vi "Subnet Mask to CIDR Prefix.vi"(7 "address":u32) -> (3 "prefix":i32)   [LabVIEW 2020, in "NI_WFCN.lvlib"]
doc: "Given a subnet mask (e.g. 255.255.255.0), returns its equivalent CIDR prefix (e.g. /24)."
uses:
  <vilib>/net/WFCN/NI_WFCN.lvlib
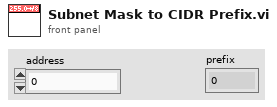
[diagram p1: front panel]
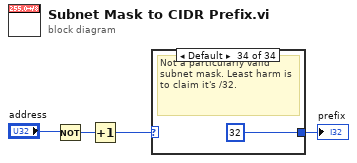
[diagram p0: block diagram]
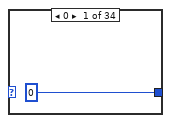
[diagram p2: hidden frame]
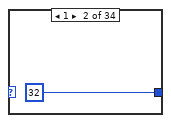
[diagram p3: hidden frame]
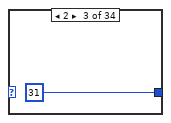
[diagram p4: hidden frame]
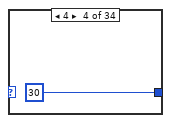
[diagram p5: hidden frame]
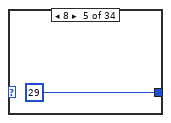
[diagram p6: hidden frame]
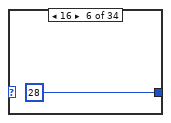
[diagram p7: hidden frame]
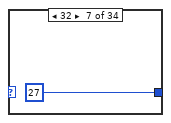
[diagram p8: hidden frame]
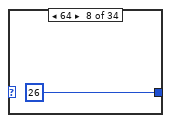
[diagram p9: hidden frame]
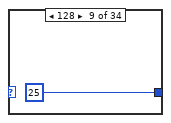
[diagram p10: hidden frame]
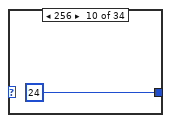
[diagram p11: hidden frame]
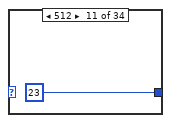
[diagram p12: hidden frame]
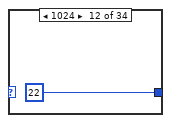
[diagram p13: hidden frame]
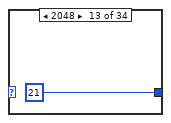
[diagram p14: hidden frame]
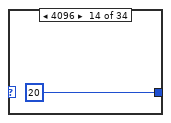
[diagram p15: hidden frame]
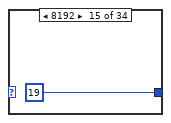
[diagram p16: hidden frame]
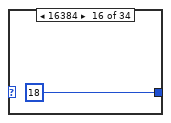
[diagram p17: hidden frame]
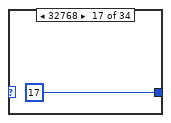
[diagram p18: hidden frame]
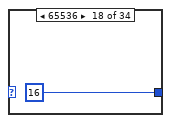
[diagram p19: hidden frame]
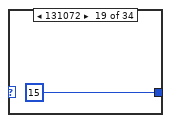
[diagram p20: hidden frame]
diagram:
  n1 = Not(x="address") -> (.not. x?=w3:u32)
  n2 = Increment(x=w3) -> (x+1=w2:u32)
  n3 = case shown="Default" w2 {
    tunnel: [0 32 31 30 29 28 27 26 25 24 23 22 21 20 19 18 17 16 15 14 13 12 11 10 9 8 7 6 5 4 3 2 1 32] -> w1
    frame 0 {
    }
    frame 1 {
    }
    frame 2 {
    }
    frame 4 {
    }
    frame 8 {
    }
    frame 16 {
    }
    frame 32 {
    }
    frame 64 {
    }
    frame 128 {
    }
    frame 256 {
    }
    frame 512 {
    }
    frame 1024 {
    }
    frame 2048 {
    }
    frame 4096 {
    }
    frame 8192 {
    }
    frame 16384 {
    }
    frame 32768 {
    }
    frame 65536 {
    }
    frame 131072 {
    }
    frame 262144 {
    }
    frame 524288 {
    }
    frame 1048576 {
    }
    frame 2097152 {
    }
    frame 4194304 {
    }
    frame 8388608 {
    }
    frame 16777216 {
    }
    frame 33554432 {
    }
    frame 67108864 {
    }
    frame 134217728 {
    }
    frame 268435456 {
    }
    frame 536870912 {
    }
    frame 1073741824 {
    }
    frame -2147483648 {
    }
    frame Default {
      # "Not a particularly valid subnet mask. Least harm is to claim it's /32."
    }
  }
  "prefix" <- w1
